vi "CISaveLoadSettings.vi"(7 "Save?":bool=TRUE, 8 "Serialized data":string, 11 "Camera data":variant) -> (0 "Serialized data (out)":string, 3 "Camera data (out)":variant)   [LabVIEW 2011]
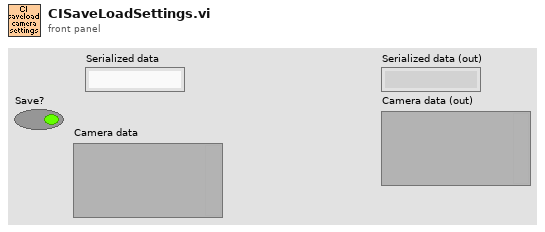
[diagram p1: front panel]
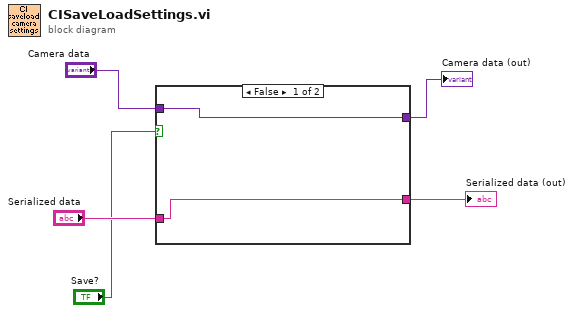
[diagram p0: block diagram]
diagram:
  n1 = case shown="False" "Save?" {
    tunnel: "Serialized data" -> [w6 w9]
    tunnel: [w6 w9] -> w4
    tunnel: [w7 w8] -> w2
    tunnel: "Camera data" -> [w7 w8]
    frame False {
    }
    frame True {
    }
  }
  "Serialized data (out)" <- w4
  "Camera data (out)" <- w2
